vi "WormQuant.vi"() -> ()   [LabVIEW 2017]
uses:
  <vilib>/Utility/file.llb/Write To Spreadsheet File (DBL).vi
  <vilib>/vision/NI_Vision_Development_Module.lvlib
panel:
  in  "Tab Control":enum32{"Instructions & Settings", "Analysis"}(tab)
  in  "Number of Wells":dbl=24.0
  out "Current Video":u8(slide) scale=0.0..151.0
  out "Overall Progress":u8(slide) scale=-1.0..70.0
  out "Full Plate":T1(plugin-control)
  in  "Threshold":dbl=7.0
  in  "Stop Updating Panel":bool
  out "path":path
  in  "Window Size (15x15)":cluster{"SizeX":i32, "SizeY":i32}={"SizeX"=15, "SizeY"=15} {"SizeY" min=3 step=1; "SizeX" min=3 step=1}
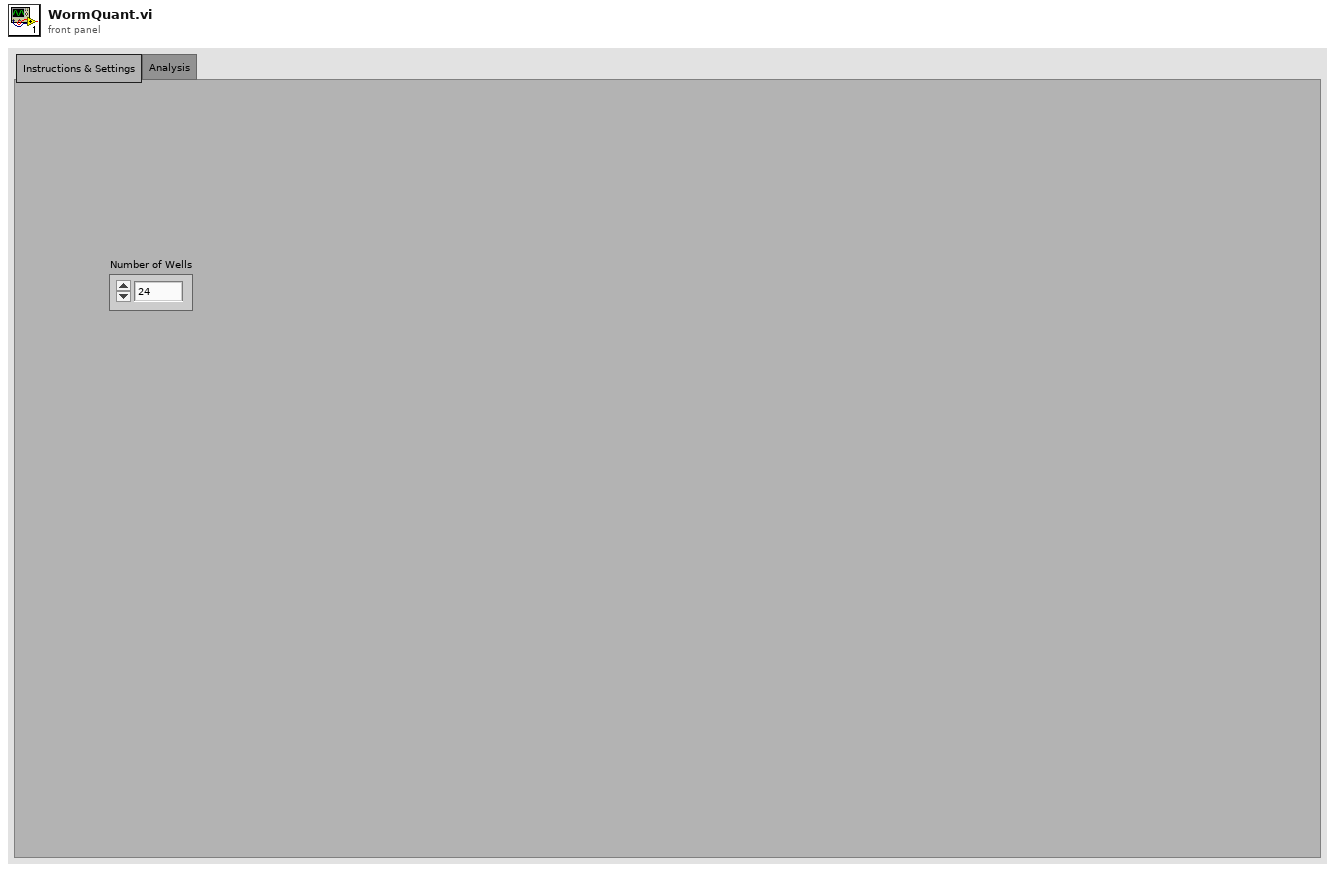
[diagram p1: front panel]
types:
  T1 = typedef "IMAQ Image.ctl" = refnum<image>
  T2 = typedef "Image Type" = u32
  T3 = typedef "IMAQ AVI2 Refnum.ctl" = refnum<k20>
  T4 = typedef "IMAQ Rectangle" = cluster{"Left":i32, "Top":i32, "Right":i32, "Bottom":i32, "Rotation":dbl}
  T5 = typedef "ROI Descriptor" = cluster{"Global Rectangle":i32[], "Contours":cluster{"ID":enum32{"External", "Internal"}, "Type":u32, "Coordinates":i32[]}[]}
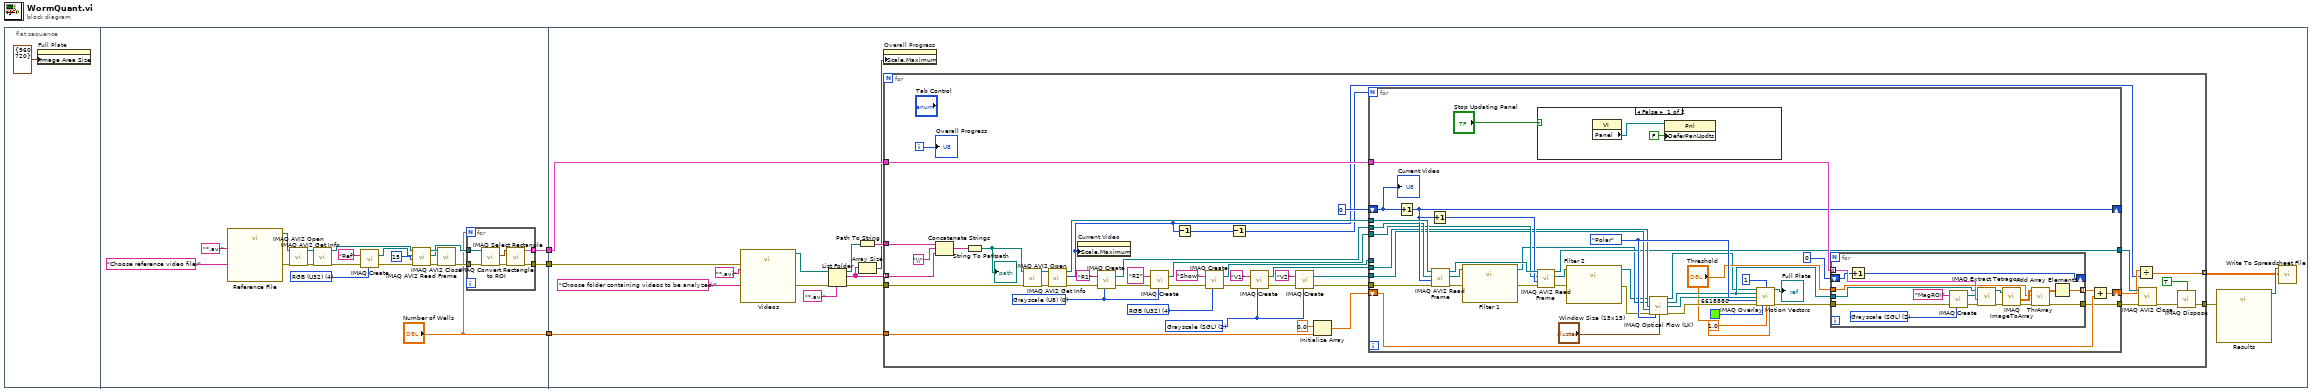
[diagram p0: block diagram]
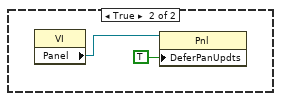
[diagram p2: hidden frame]
diagram:
  n1 = flat-sequence {
    tunnel: [w7] -> w3
    tunnel: [w6] -> w2
    tunnel: ["Number of Wells"] -> w1
    tunnel: w3 -> [w46]
    tunnel: w2 -> [w45]
    tunnel: w1 -> [w42]
    frame #0 {
      n2 = property on="Full Plate" class="ImageControl"("Image Area Size"=cluster{"Width":u32, "Height":u32} {"Width"=960, "Height"=720} ("Image Area:Size:All Elements")) -> ()  [unwired: 2 in, 2 out]
    }
    frame #1 {
      w19 = T2 4 items=["Grayscale (U8)", "Grayscale (I16)", "Grayscale (SGL)", "Complex (CSG)", "RGB (U32)", "HSL (U32)", "RGB (U64)", "Grayscale (U16)"] ("Image Type")
      n3 = call "Reference File"("prompt"="Choose reference video file:", "pattern (all files)"="*.avi") -> ("selected path"=w12:path, "error out"=w13:errorcluster)  [unwired: 10 in, 2 out]
      n4 = call "IMAQ AVI2 Open"("error in (no error)"=w13, "AVI File Path"=w12) -> ("error out"=w10:errorcluster, "AVI Refnum"=w11:T3)  [unwired: 8 in]
      n5 = call "IMAQ AVI2 Get Info"("error in (no error)"=w10, "AVI Refnum"=w11) -> ("error out"=w15:errorcluster, "AVI Refnum (duplicate)"=w14:T3)  [unwired: 5 in, 3 out]
      n6 = call "IMAQ Create"("Image Name"="Ref", "Image Type"=w19, "error in (no error)"=w15) -> ("New Image"=w17:T1, "error out"=w16:errorcluster)  [unwired: 2 in]
      n7 = call "IMAQ AVI2 Read Frame"("error in (no error)"=w16, "Frame Number"=u32 15, "Image"=w17, "AVI Refnum"=w14) -> ("error out"=w23:errorcluster, "Image Out"=w20:T1, "AVI Refnum (duplicate)"=w22:T3)  [unwired: 5 in]
      n8 = call "IMAQ AVI2 Close"("error in (no error)"=w23, "AVI Refnum"=w22) -> ("error out"=w24:errorcluster)  [unwired: 9 in]
      n9 = for {
        N: "Number of Wells" -> [_]
        tunnel: w20 -> [w30]
        tunnel: [w27] -> w6
        tunnel: w24 -> [w26]
        tunnel: [w25] -> w7 mode=indexing
        n10 = call "IMAQ Select Rectangle"("error in (no error)"=w26, "Image In"=w30) -> ("error out"=w28:errorcluster, "Rectangle"=w29:T4)  [unwired: 6 in, 2 out]
        n11 = call "IMAQ Convert Rectangle to ROI"("error in (no error)"=w28, "Rectangle"=w29) -> ("error out"=w27:errorcluster, "ROI Descriptor"=w25:T5)  [unwired: 7 in]
      }
    }
    frame #2 {
      n12 = call "Videos"("prompt"="Choose folder containing videos to be analyzed:", "error in"=w45, "pattern (all files)"="*.avi" ("pattern")) -> ("selected path"=w39:path, "error out"=w38:errorcluster)  [unwired: 9 in, 2 out]
      n13 = List Folder(path=w39, pattern="*.avi", error in=w38) -> (path out=w41:path, filenames=w33:string[], error out=w36:errorcluster)  [unwired: 1 in, 1 out]
      n14 = Path To String(path=w41) -> (string=w37:string)
      n15 = Array Size(array=w33) -> (size(s)=w32:i32)
      n16 = property on="Overall Progress" class="Slide (strict)"("Scale.Maximum"=w32) -> ()  [unwired: 2 in, 2 out]
      n17 = for {
        tunnel: w46 -> [w84]
        tunnel: [w69] -> w31 mode=indexing
        tunnel: w42 -> [w81]
        tunnel: [w66] -> w44
        tunnel: w37 -> [w76]
        tunnel: w33 -> [w75] mode=indexing
        tunnel: w36 -> [w74]
        i -> [w72]
        w47 = T2 4 items=["Grayscale (U8)", "Grayscale (I16)", "Grayscale (SGL)", "Complex (CSG)", "RGB (U32)", "HSL (U32)", "RGB (U64)", "Grayscale (U16)"] ("Image Type")
        w49 = T2 2 items=["Grayscale (U8)", "Grayscale (I16)", "Grayscale (SGL)", "Complex (CSG)", "RGB (U32)", "HSL (U32)", "RGB (U64)", "Grayscale (U16)"] ("Image Type")
        w60 = T2 0 items=["Grayscale (U8)", "Grayscale (I16)", "Grayscale (SGL)", "Complex (CSG)", "RGB (U32)", "HSL (U32)", "RGB (U64)", "Grayscale (U16)"] ("Image Type")
        n18 = Concatenate Strings(w76, "\\" ("string"), w75) -> (w77:string)
        n19 = String To Path(string=w77) -> (path=w73:path)
        "path" <- w73
        n20 = call "IMAQ AVI2 Open"("error in (no error)"=w74, "AVI File Path"=w73) -> ("error out"=w85:errorcluster, "AVI Refnum"=w86:T3)  [unwired: 8 in]
        n21 = call "IMAQ AVI2 Get Info"("error in (no error)"=w85, "AVI Refnum"=w86) -> ("error out"=w64:errorcluster, "Number of Frames"=w70:u32, "AVI Refnum (duplicate)"=w87:T3)  [unwired: 5 in, 2 out]
        n22 = property on="Current Video" class="Slide (strict)"("Scale.Maximum"=w70) -> ()  [unwired: 2 in, 2 out]
        n23 = call "IMAQ Create"("Image Name"="R1", "Image Type"=w60, "error in (no error)"=w64) -> ("New Image"=w63:T1, "error out"=w61:errorcluster)  [unwired: 2 in]
        n24 = call "IMAQ Create"("Image Name"="R2", "Image Type"=w60, "error in (no error)"=w61) -> ("New Image"=w59:T1, "error out"=w56:errorcluster)  [unwired: 2 in]
        n25 = Decrement(x=w70) -> (x-1=w82:u32)
        n26 = call "IMAQ Create"("Image Name"="Show", "Image Type"=w47, "error in (no error)"=w56) -> ("New Image"=w57:T1, "error out"=w53:errorcluster)  [unwired: 2 in]
        n27 = Decrement(x=w82) -> (x-1=w83:u32)
        n28 = call "IMAQ Create"("Image Name"="V1", "Image Type"=w49, "error in (no error)"=w53) -> ("New Image"=w54:T1, "error out"=w51:errorcluster)  [unwired: 2 in]
        n29 = call "IMAQ Create"("Image Name"="V2", "Image Type"=w49, "error in (no error)"=w51) -> ("New Image"=w50:T1, "error out"=w48:errorcluster)  [unwired: 2 in]
        n30 = Initialize Array(sgl 0.0 ("element"), w81) -> (w79:sgl[])
        n31 = for {
          N: w83 -> [_]
          tunnel: w87 -> [w128]
          tunnel: [w110] -> w88
          tunnel: [w99] -> w89
          shift-right: [w116] -> _
          shift-left: 0 -> [w111]
          tunnel: w84 -> [w124]
          shift-right: [w118] -> w71
          shift-left: w79 -> [w120]
          tunnel: w63 -> [w109]
          tunnel: w59 -> [w108]
          tunnel: w57 -> [_]
          tunnel: w54 -> [w107]
          tunnel: w50 -> [w106]
          tunnel: w48 -> [w105]
          w123 = enum16{"Cartesian", "Polar"}."Polar" ("Velocity Representation")
          n32 = Increment(x=w111) -> (x+1=w116:i32)
          n33 = Increment(x=w116) -> (x+1=w113:i32)
          n34 = call "IMAQ AVI2 Read Frame"("error in (no error)"=w105, "Frame Number"=w116, "Image"=w109, "AVI Refnum"=w128) -> ("error out"=w96:errorcluster, "Image Out"=w98:T1, "AVI Refnum (duplicate)"=w127:T3)  [unwired: 5 in]
          n35 = call "Filter 1"("Image In"=w98, "error in"=w96) -> ("Image Out"=w97:T1, "error out"=w95:errorcluster)  [unwired: 24 in]
          n36 = case shown="False" "Stop Updating Panel" {
            frame False {
              n37 = property class="VI"() -> ("Panel"=w129:refnum<vi>)  [unwired: 2 in, 2 out]
              n38 = property class="Pnl"(reference=w129, "DeferPanUpdts"=FALSE ("Defer Panel Updates")) -> ()  [unwired: 1 in, 2 out]
            }
            frame True {
              n39 = property class="VI"() -> ("Panel"=w131:refnum<vi>)  [unwired: 2 in, 2 out]
              n40 = property class="Pnl"(reference=w131, "DeferPanUpdts"=TRUE ("Defer Panel Updates")) -> ()  [unwired: 1 in, 2 out]
            }
          }
          n41 = call "IMAQ AVI2 Read Frame"("error in (no error)"=w95, "Frame Number"=w113, "Image"=w108, "AVI Refnum"=w127) -> ("error out"=w94:errorcluster, "Image Out"=w92:T1, "AVI Refnum (duplicate)"=w99:T3)  [unwired: 5 in]
          n42 = call "Filter 2"("Image In"=w92, "error in"=w94) -> ("Image Out"=w91:T1, "error out"=w93:errorcluster)  [unwired: 24 in]
          n43 = call "IMAQ Optical Flow (LK)"("Current Frame"=w91, "Previous Frame"=w97, "Velocity Component 1 In"=w107, "Velocity Component 2 In"=w106, "error in (no error)"=w93, "Velocity Representation"=w123, "Window Size (15x15)"="Window Size (15x15)") -> ("Current Frame Out (dup)"=w100:T1, "Velocity Component 1 Out"=w122:T1, "Velocity Component 2 Out"=w125:T1, "error out"=w126:errorcluster)  [unwired: 5 in]
          n44 = call "IMAQ Overlay Motion Vectors"("Image"=w100, "Step Size"=1, "Velocity Component 1"=w122, "Velocity Component 2"=w125, "Velocity Representation"=w123, "error in (no error)"=w126, "Color"=u32 6618880, "Scale"=1.0, "Threshold"="Threshold") -> ("Image Out"=→"Full Plate":T1, "error out"=w121:errorcluster)  [unwired: 5 in]
          n45 = for {
            tunnel: w124 -> [w149] mode=indexing
            tunnel: w122 -> [w148]
            tunnel: w121 -> [w142]
            tunnel: [w141] -> w119 mode=indexing
            tunnel: "Threshold" -> [w137]
            shift-right: [w139] -> _
            shift-left: 0 -> [w140]
            tunnel: [w133] -> w110
            w134 = T2 2 items=["Grayscale (U8)", "Grayscale (I16)", "Grayscale (SGL)", "Complex (CSG)", "RGB (U32)", "HSL (U32)", "RGB (U64)", "Grayscale (U16)"] ("Image Type")
            n46 = Increment(x=w140) -> (x+1=w139:i32)
            n47 = call "IMAQ Create"("Image Name"="MagROI", "Image Type"=w134, "error in (no error)"=w142) -> ("New Image"=w146:T1, "error out"=w147:errorcluster)  [unwired: 2 in]
            n48 = call-poly "IMAQ Extract Tetragon"("error in (no error)"=w147, "ROI Descriptor"=w149, "Image Dst"=w146, "Image Src"=w148) -> ("error out"=w144:errorcluster, "Image Dst Out"=w143:T1)  [unwired: 6 in]
            n49 = call "IMAQ ImageToArray"("error in (no error)"=w144, "Image"=w143) -> ("Image Pixels (Float)"=w138:sgl[][], "error out"=w135:errorcluster)  [unwired: 2 in, 3 out]
            n50 = call "ThrArray.vi"("Error In"=w135, "Threshold"=w137, "Input Array"=w138) -> ("Error Out"=w133:errorcluster, "Array"=w136:dbl[][])  [unwired: 7 in]
            n51 = Add Array Elements(numeric array=w136) -> (sum=w141:dbl)
          }
          n52 = Add(x=w119, y=w120) -> (x+y=w118:dbl[])
          "Current Video" <- w111
        }
        n53 = Divide(x=w71, y=w70) -> (x/y=w69:dbl[])
        n54 = call "IMAQ AVI2 Close"("error in (no error)"=w88, "AVI Refnum"=w89) -> ("error out"=w67:errorcluster)  [unwired: 9 in]
        n55 = call "IMAQ Dispose"("All Images? (No)"=TRUE, "error in (no error)"=w67) -> ("error out"=w66:errorcluster)  [unwired: 4 in]
        "Overall Progress" <- w72
      }
      n56 = call "Results"("error in"=w44) -> ("selected path"=w43:path)  [unwired: 11 in, 3 out]
      n57 = call-poly <vilib>:"Write To Spreadsheet File.vi"("2D data"=w31, "file path (dialog if empty)"=w43) -> ()  [unwired: 6 in, 1 out]
    }
  }
